vi "load_driver_and_panel.vi"(4 "error in (no error)":errorcluster, 6 "VIpath":path, 7 "Sub Panel in":refnum<vi>) -> (0 "error out":errorcluster, 2 "driver VI Refnum":refnum<vi>, 3 "Sub Panel out":refnum<vi>)   [LabVIEW 2010]
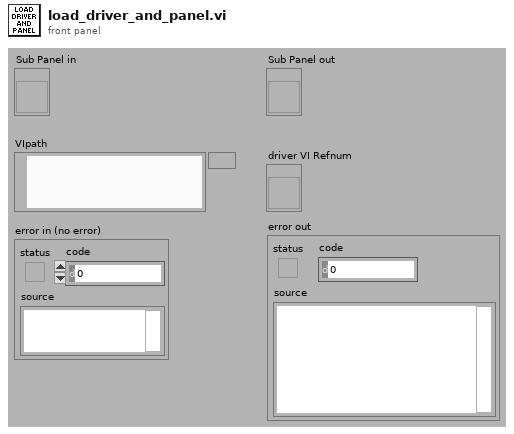
[diagram p1: front panel]
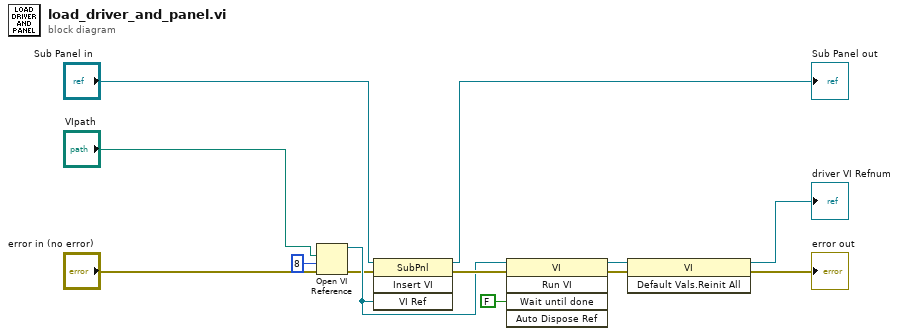
[diagram p0: block diagram]
diagram:
  n1 = Open VI Reference(vi path="VIpath", options=8, error in (no error)="error in (no error)") -> (vi reference=w11:refnum<vi>, error out=w10:errorcluster)  [unwired: 3 in]
  n2 = invoke class="SubPnl" method="Insert VI"(reference="Sub Panel in", error in=w10, "VI Ref"=w11) -> (reference out=→"Sub Panel out":refnum<vi>, error out=w12:errorcluster)  [unwired: 1 in, 2 out]
  n3 = invoke class="VI" method="Run VI"(reference=w11, error in=w12, "Wait until done"=FALSE ("Wait Until Done")) -> (reference out=w4:refnum<vi>, error out=w3:errorcluster)  [unwired: 2 in, 3 out]
  n4 = invoke class="VI" method="Default Vals.Reinit All"(reference=w4, error in=w3) -> (reference out=→"driver VI Refnum":refnum<vi>, error out=→"error out":errorcluster)  [unwired: 1 in, 1 out]
